vi "R.vi"(6 "ID(Hex 高位有效)":string="312", 7 "通信协议名称":string, 8 "错误输入（无错误）":errorcluster, 9 "DelayTime":u32=1000, 10 "CANChannel":u32, 11 "VISA资源名称":refnum<visa-resource-name>="COM1") -> (0 "错误输出":errorcluster, 1 "VCI_CAN_OBJ_R":T1 {"ID" format="%x"}, 2 "CMD":string)   [LabVIEW 2013]
uses:
  InitConfig.ctl
  DevType.ctl
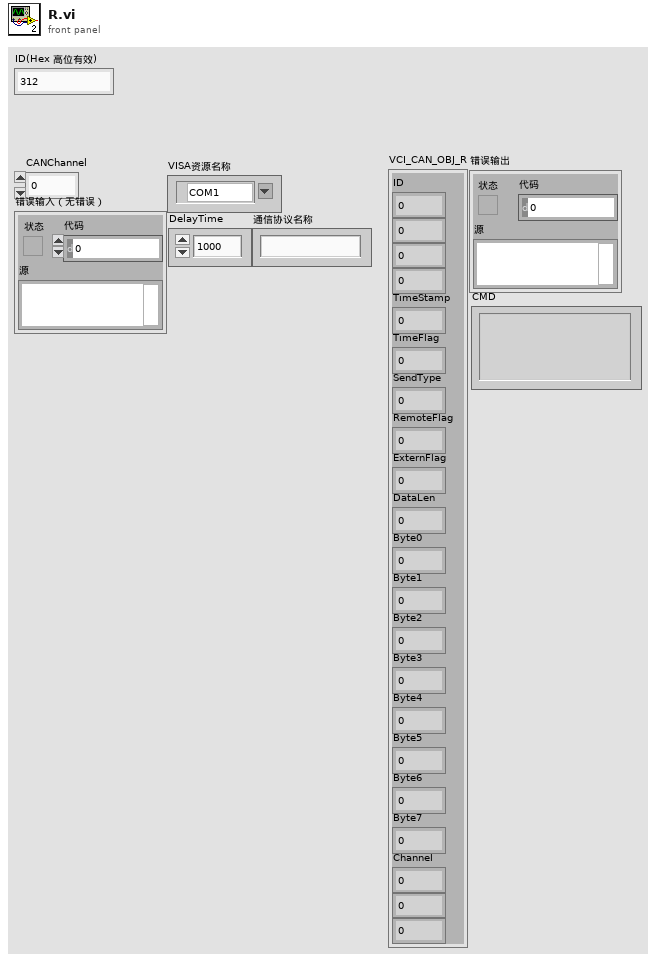
[diagram p1: front panel]
types:
  T1 = cluster{"ID":u8, u8, u8, u8, "TimeStamp":u32, "TimeFlag":u8, "SendType":u8, "RemoteFlag":u8, "ExternFlag":u8, "DataLen":u8, "Byte0":u8, "Byte1":u8, "Byte2":u8, "Byte3":u8, "Byte4":u8, "Byte5":u8, "Byte6":u8, "Byte7":u8, "Channel":u8, u8, u8}
  T2 = typedef "DevType.ctl" = u16
  T3 = typedef "InitConfig.ctl" = cluster{"AccCode":u32, "AccMask":u32, "Reserved":u32, "Filter":u8, "kCanBaud":u8, "Timing0":u8, "Timing1":u8, "Mode":u8, "CanRx_IER":u8}
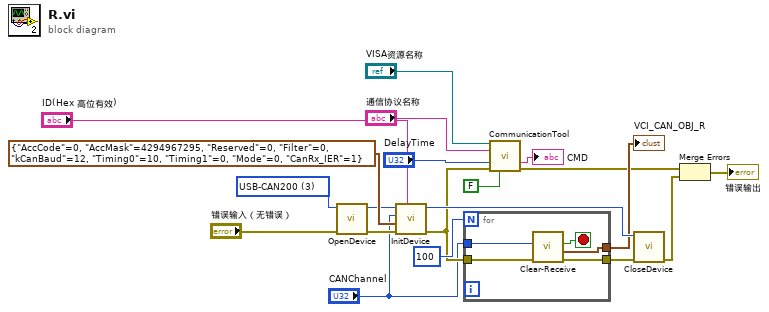
[diagram p0: block diagram]
diagram:
  w18 = T2 3 items=["PCI-CAN200"=7, "USB-CAN"=2, "USB-CAN200"=3] ("DeviceType")
  n1 = call "OpenDevice.vi"("错误输入（无错误）"="错误输入（无错误）", "DeviceType"=w18) -> ("错误输出"=w17:errorcluster, "DeviceTypeOut"=w19:u16)  [unwired: 7 in, 1 out]
  n2 = call "InitDevice.vi"("ID(Hex 高位有效)"="ID(Hex 高位有效)", "错误输入（无错误）"=w17, "InitConfig"=T3 {"AccCode"=0, "AccMask"=4294967295, "Reserved"=0, "Filter"=0, "kCanBaud"=12, "Timing0"=10, "Timing1"=0, "Mode"=0, "CanRx_IER"=1}, "CanChannel"="CANChannel", "DeviceType"=w19) -> ("错误输出"=w10:errorcluster, "DeviceTypeOut"=w14:u16)  [unwired: 4 in, 1 out]
  n3 = for {
    N: 100 -> [_]
    tunnel: "CANChannel" -> [w25]
    tunnel: w10 -> [w24]
    tunnel: [w22] -> w13
    tunnel: [w21] -> w15
    stop <- w23 stop-if-true
    n4 = call "Clear-Receive.vi"("错误输入（无错误）"=w24, "CANChannel"=w25) -> ("错误输出"=w21:errorcluster, "VCI_CAN_OBJ_R"=w22:T1, "Result"=w23:bool)  [unwired: 3 in, 4 out]
  }
  "VCI_CAN_OBJ_R" <- w13
  n5 = call "CommunicationTool.vi"("VISA资源名称"="VISA资源名称", "通信协议名称"="通信协议名称", "DelayTime"="DelayTime", "error in"=w10, "Debug"=FALSE) -> ("CMD"=→"CMD":string, "error out"=w9:errorcluster)  [unwired: 5 in, 4 out]
  n6 = call "CloseDevice.vi"("错误输入（无错误）"=w15, "DeviceType"=w14) -> ("错误输出"=w8:errorcluster)  [unwired: 7 in, 2 out]
  n7 = Merge Errors(w9, w8) -> (→"错误输出":errorcluster)
